vi "Init.vi"(8 "error in (no error)":errorcluster, 10 "Stream":refnum<class "Stream.lvclass">) -> (0 "error out":errorcluster, 3 "FormulaG API out":refnum<class "FormulaG API.lvclass">)   [LabVIEW 2020, in "FormulaG.lvlib" / "FormulaG API.lvclass"]
uses:
  FormulaG API.lvclass
  <vilib>/IlluminatedG/lv-stream/stream/Stream.lvclass
  <vilib>/IlluminatedG/IG WebSocket Stream/Stream-Websocket/WebsocketStream/WebsocketStream.lvclass
  FormulaG API.lvclass/FormulaG API.ctl
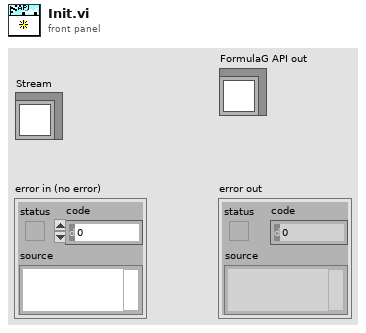
[diagram p1: front panel]
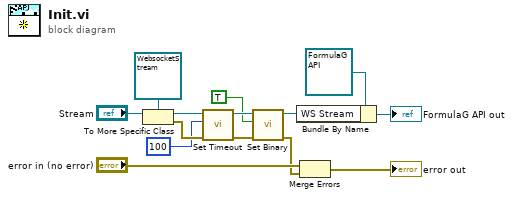
[diagram p0: block diagram]
diagram:
  n1 = To More Specific Class(target class=refnum<class "WebsocketStream.lvclass"> refnum ("WebsocketStream in"), reference="Stream") -> (specific class reference=w5:refnum<class "WebsocketStream.lvclass">, error out=w14:errorcluster)  [unwired: 1 in]
  n2 = call <vilib>:"Set Timeout.vi"("error in (no error)"=w14, "Timeout ms"=100, "WebsocketStream in"=w5) -> ("error out"=w3:errorcluster, "WebsocketStream out"=w10:refnum<class "WebsocketStream.lvclass">)  [unwired: 7 in]
  n3 = call <vilib>:"Set Binary.vi"("error in (no error)"=w3, "Binary"=TRUE, "WebsocketStream in"=w10) -> ("error out"=w1:errorcluster, "WebsocketStream out"=w7:refnum<class "WebsocketStream.lvclass">)  [unwired: 7 in]
  n4 = Bundle By Name(cluster=refnum<class "FormulaG API.lvclass"> refnum ("FormulaG API in"), "WS Stream"=w7) -> (→"FormulaG API out":refnum<class "FormulaG API.lvclass">)
  n5 = Merge Errors("error in (no error)", w1) -> (→"error out":errorcluster)
